vi "gate current sweep.vi"() -> ()   [LabVIEW 2010]
uses:
  <vilib>/Utility/file.llb/Write To Spreadsheet File (DBL).vi
  <userlib>/Nanonis Prog Interface V5/Nanonis Prog Interface.lvlib
panel:
  in  "Plot Current or Z?":bool=TRUE
  out "XY Graph":cluster{dbl[], sgl[]}(graph)
  in  "Number of Z Averages":i32=1
  in  "Number of Current Averages":i32=20
  out "Current Gate Voltage (V)":dbl
  in  "Increment Gate (V)":dbl
  in  "End Gate (V)":dbl
  in  "Start Gate (V)":dbl
  in  "Filename":string
  # "Gate-Current Sweep"
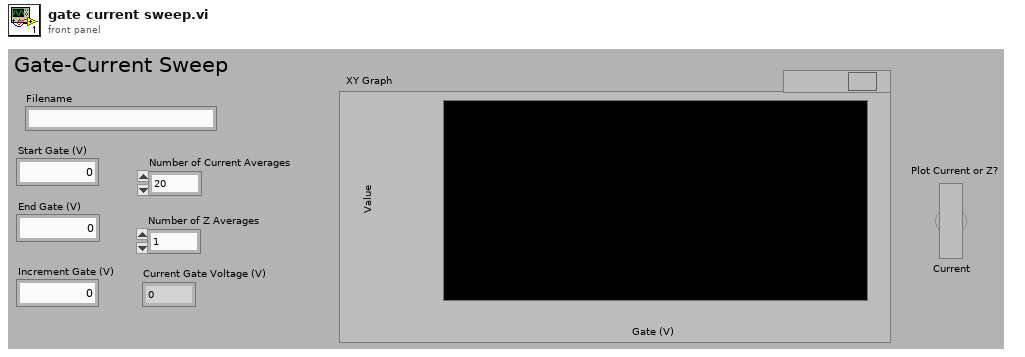
[diagram p1: front panel]
types:
  T1 = enum16{"Set Voltage", "Read Voltage", "Read Setpoint", "Read Current", "Output On", "Output Off"}
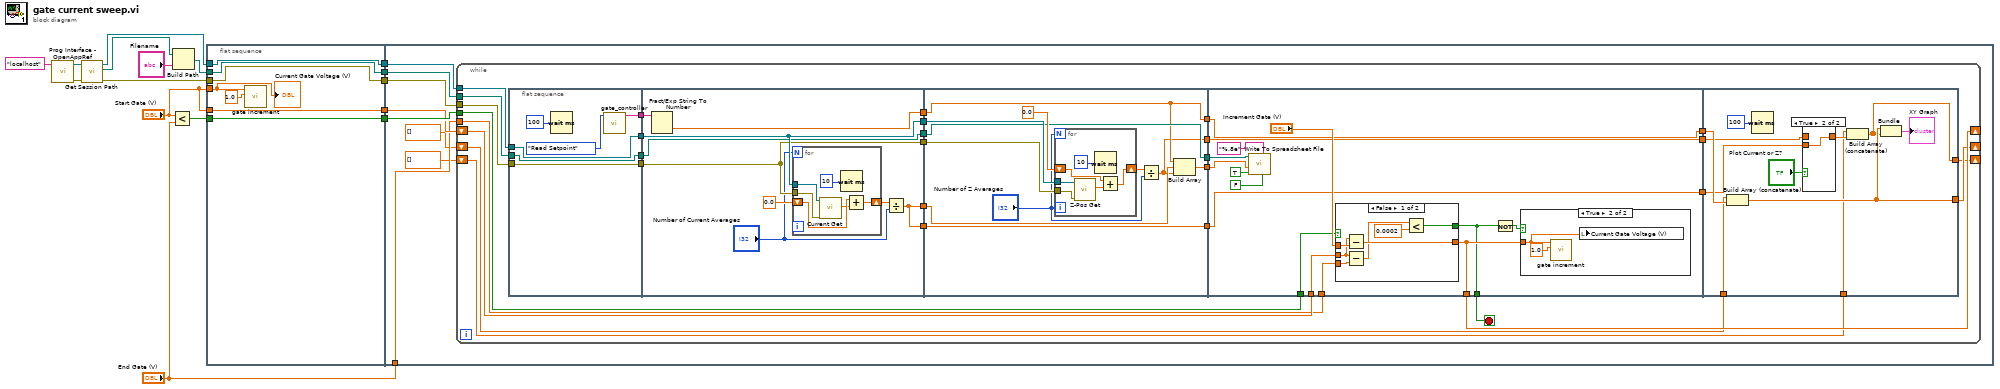
[diagram p0: block diagram]
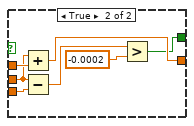
[diagram p2: hidden frame]
diagram:
  n1 = call <userlib>:"Prog Interface - OpenAppRef.vi"("Machine name (local machine IP)"="localhost" ("machine name (localhost)")) -> ("Error out"=w7:errorcluster, "Application reference"=w8:refnum<vi>)  [unwired: 5 in]
  n2 = call <userlib>:"Get Session Path.vi"("error in (no error)"=w7, "Application ref in"=w8) -> ("error out"=w6:errorcluster, "Session path"=w4:path, "Application ref out"=w5:refnum<vi>)  [unwired: 7 in]
  n3 = Less?(x="Start Gate (V)", y="End Gate (V)") -> (x < y?=w15:bool)
  n4 = Build Path(base path=w4, name or relative path="Filename") -> (appended path=w2:path)
  n5 = flat-sequence {
    tunnel: "Start Gate (V)" -> [w20]
    tunnel: w15 -> [w21]
    tunnel: w5 -> [w22]
    tunnel: w6 -> [w23]
    tunnel: [w23] -> w14
    tunnel: [w22] -> w13
    tunnel: [w21] -> w12
    tunnel: [w20] -> w11
    tunnel: "Start Gate (V)" -> [w18]
    tunnel: w2 -> [w17]
    tunnel: [w17] -> w1
    tunnel: w14 -> [w31]
    tunnel: w13 -> [w30]
    tunnel: w12 -> [w29]
    tunnel: w11 -> [w28]
    tunnel: "End Gate (V)" -> [w27]
    tunnel: w1 -> [w26]
    frame #0 {
      n6 = call "gate increment.vi"("Increment"=1.0, "Gate Voltage"=w18) -> ()  [unwired: 10 in]
      "Current Gate Voltage (V)" <- w18
    }
    frame #1 {
      n7 = while {
        tunnel: w31 -> [w61]
        tunnel: w30 -> [w60]
        tunnel: w29 -> [w54]
        shift-right: [w57] -> _
        shift-left: w28 -> [w56]
        tunnel: w27 -> [w55]
        tunnel: w26 -> [w46]
        shift-right: [w40] -> _
        shift-left: dbl[] [] -> [w39]
        shift-right: [w33] -> _
        shift-left: sgl[] [] -> [w32]
        stop <- w53 stop-if-true
        n8 = flat-sequence {
          tunnel: w60 -> [w66]
          tunnel: w61 -> [w67]
          tunnel: [w67] -> w59
          tunnel: [w66] -> w58
          tunnel: [w63] -> w50
          tunnel: w46 -> [w62]
          tunnel: [w62] -> w43
          tunnel: w59 -> [w74]
          tunnel: w58 -> [w75]
          tunnel: [w75] -> w52
          tunnel: [w74] -> w51
          tunnel: w50 -> [w71]
          tunnel: [w70] -> w49
          tunnel: [w68] -> w48
          tunnel: [w69] -> w44
          tunnel: w43 -> [w69]
          tunnel: [w68] -> w36
          tunnel: w52 -> [w92]
          tunnel: w51 -> [w91]
          tunnel: w49 -> [w85]
          tunnel: w48 -> [w88]
          tunnel: [w87] -> w47
          tunnel: [w86] -> w45
          tunnel: w44 -> [w86]
          tunnel: [w85] -> w42
          tunnel: [w84] -> w37
          tunnel: w36 -> [w84]
          tunnel: [w83] -> w34
          tunnel: [w114] -> w57
          tunnel: [w113] -> w53
          tunnel: w56 -> [w112]
          tunnel: w55 -> [w110]
          tunnel: w54 -> [w109]
          tunnel: w47 -> [w105]
          tunnel: w45 -> [w104]
          tunnel: w42 -> [w102]
          tunnel: [w102] -> w41
          tunnel: [w101] -> w38
          tunnel: w37 -> [w101]
          tunnel: [w100] -> w35
          tunnel: w34 -> [w100]
          tunnel: w41 -> [w139]
          tunnel: [w138] -> w40
          tunnel: w39 -> [w137]
          tunnel: w38 -> [w135]
          tunnel: w35 -> [w134]
          tunnel: [w132] -> w33
          tunnel: w32 -> [w131]
          frame #0 {
            n9 = Wait (ms)(milliseconds to wait=u32 100) -> ()  [unwired: 1 out]
            n10 = call "gate_controller.vi"("Command"=T1."Read Setpoint") -> ("Response"=w63:string)  [unwired: 10 in]
          }
          frame #1 {
            n11 = Fract/Exp String To Number(string=w71) -> (number=w70:dbl)  [unwired: 3 in, 1 out]
            n12 = for {
              N: "Number of Current Averages" -> [_]
              tunnel: w75 -> [w82]
              tunnel: w74 -> [w81]
              shift-right: [w80] -> w73
              shift-left: sgl 0.0 ("Current (A)") -> [w79]
              n13 = call <userlib>:"Current Get.vi"("Error in (no error)"=w81, "Application ref in"=w82) -> ("Current (A)"=w78:sgl)  [unwired: 5 in, 2 out]
              n14 = Wait (ms)(milliseconds to wait=u32 10) -> ()  [unwired: 1 out]
              n15 = Add(x=w79, y=w78) -> (x+y=w80:sgl)
            }
            n16 = Divide(x=w73, y="Number of Current Averages") -> (x/y=w68:sgl)
          }
          frame #2 {
            n17 = for {
              N: "Number of Z Averages" -> [_]
              tunnel: w92 -> [w96]
              tunnel: w91 -> [w97]
              shift-right: [w99] -> w90
              shift-left: sgl 0.0 ("Current (A)") -> [w98]
              n18 = call <userlib>:"Z-Pos Get.vi"("error in (no error)"=w97, "Application ref in"=w96) -> ("Z position (m)"=w95:sgl)  [unwired: 7 in, 2 out]
              n19 = Wait (ms)(milliseconds to wait=u32 10) -> ()  [unwired: 1 out]
              n20 = Add(x=w98, y=w95) -> (x+y=w99:sgl)
            }
            n21 = Divide(x=w90, y="Number of Z Averages") -> (x/y=w83:sgl)
            n22 = Build Array(w85, w88, w83) -> (w87:dbl[])
          }
          frame #3 {
            n23 = call-poly <vilib>:"Write To Spreadsheet File.vi"("transpose? (no:F)"=FALSE, "format (%.3f)"="%.8e", "append to file? (new file:F)"=TRUE, "1D data"=w105, "file path (dialog if empty)"=w104) -> ()  [unwired: 3 in, 1 out]
            n24 = case shown="False" w109 {
              tunnel: w112 -> [w119 w125]
              tunnel: "Increment Gate (V)" -> [w120 w128]
              tunnel: [w121 w127] -> w114
              tunnel: w110 -> [w118 w126]
              tunnel: [w116 w124] -> w113
              frame False {
                n25 = Subtract(x=w119, y=w120) -> (x-y=w121:dbl)
                n26 = Subtract(x=w119, y=w118) -> (x-y=w117:dbl)
                n27 = Less?(x=w117, y=0.0002) -> (x < y?=w116:bool)
              }
              frame True {
                n28 = Add(x=w125, y=w128) -> (x+y=w127:dbl)
                n29 = Subtract(x=w125, y=w126) -> (x-y=w123:dbl)
                n30 = Greater?(x=w123, y=-0.0002) -> (0:w124:bool)
              }
            }
            n31 = Not(x=w113) -> (.not. x?=w108:bool)
            n32 = case shown="True" w108 {
              tunnel: w114 -> [_ w130]
              frame False {
              }
              frame True {
                n33 = call "gate increment.vi"("Increment"=1.0, "Gate Voltage"=w130) -> ()  [unwired: 10 in]
                n34 = local write "Current Gate Voltage (V)"(w130) -> ()
              }
            }
          }
          frame #4 {
            n35 = Build Array (concatenate)(w137, w139) -> (w138:dbl[])
            n36 = Wait (ms)(milliseconds to wait=u32 100) -> ()  [unwired: 1 out]
            n37 = case shown="True" "Plot Current or Z?" {
              tunnel: w135 -> [_ w143]
              tunnel: [w142 w143] -> w133
              tunnel: w134 -> [w142 _]
              frame False {
              }
              frame True {
              }
            }
            n38 = Build Array (concatenate)(w131, w133) -> (w132:sgl[])
            n39 = Bundle(w138, w132) -> (→"XY Graph":cluster{dbl[], sgl[]})  [unwired: 1 in]
          }
        }
      }
    }
  }
